vi "DC Voltage Source (Express).vi"() -> ()   [LabVIEW 2015]
panel:
  out "error out":errorcluster
  in  "stop":bool
  in  "Voltage":dbl
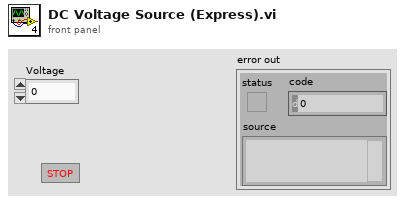
[diagram p1: front panel]
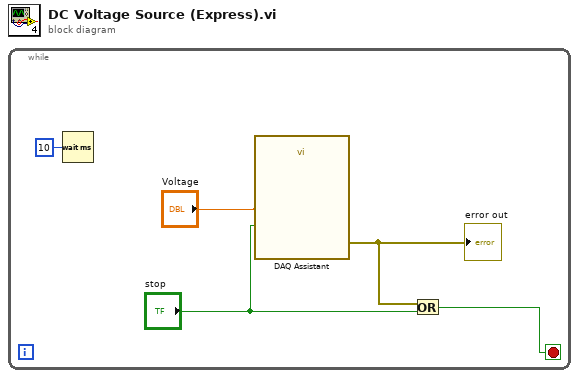
[diagram p0: block diagram]
diagram:
  n1 = while {
    stop <- w1 stop-if-true
    n2 = Wait (ms)(milliseconds to wait=u32 10) -> ()  [unwired: 1 out]
    n3 = call "DAQ Assistant"("data"="Voltage", "stop (T)"="stop") -> ("error out"=w3:errorcluster)  [unwired: 16 in, 1 out]
    "error out" <- w3
    n4 = Or(x=w3, y="stop") -> (x .or. y?=w1:bool)
  }
